vi "数字麦克风信号解析.vi"() -> ()   [LabVIEW 2024]
panel:
  in  "数值 2":i32=1
  out "长度":i32
  in  "数值":i32=400000
  out "文本":string
  out "波形图":i32[](graph)
  in  "路径":path=path "D:/Labviewworks/数字麦克风信号解析/采集数据文件/6060.log"
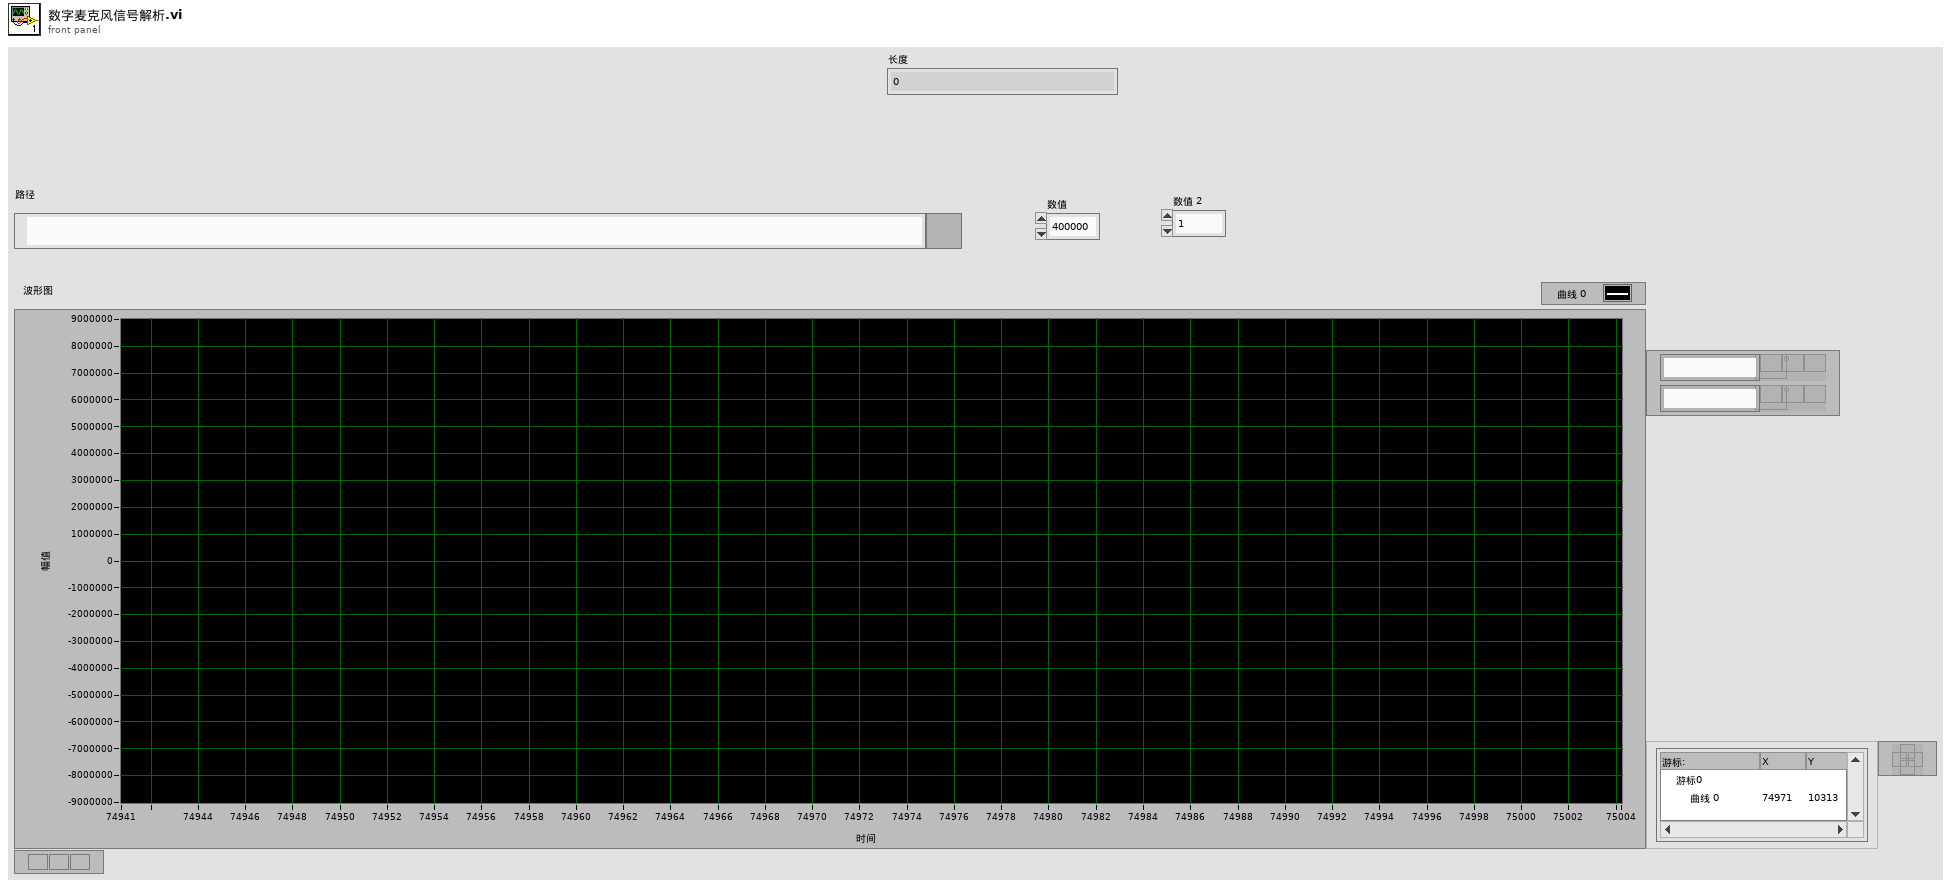
[diagram p1: front panel]
types:
  T1 = enum16{"open", "replace", "create", "open or create", "replace or create", "replace or create with confirmation"}
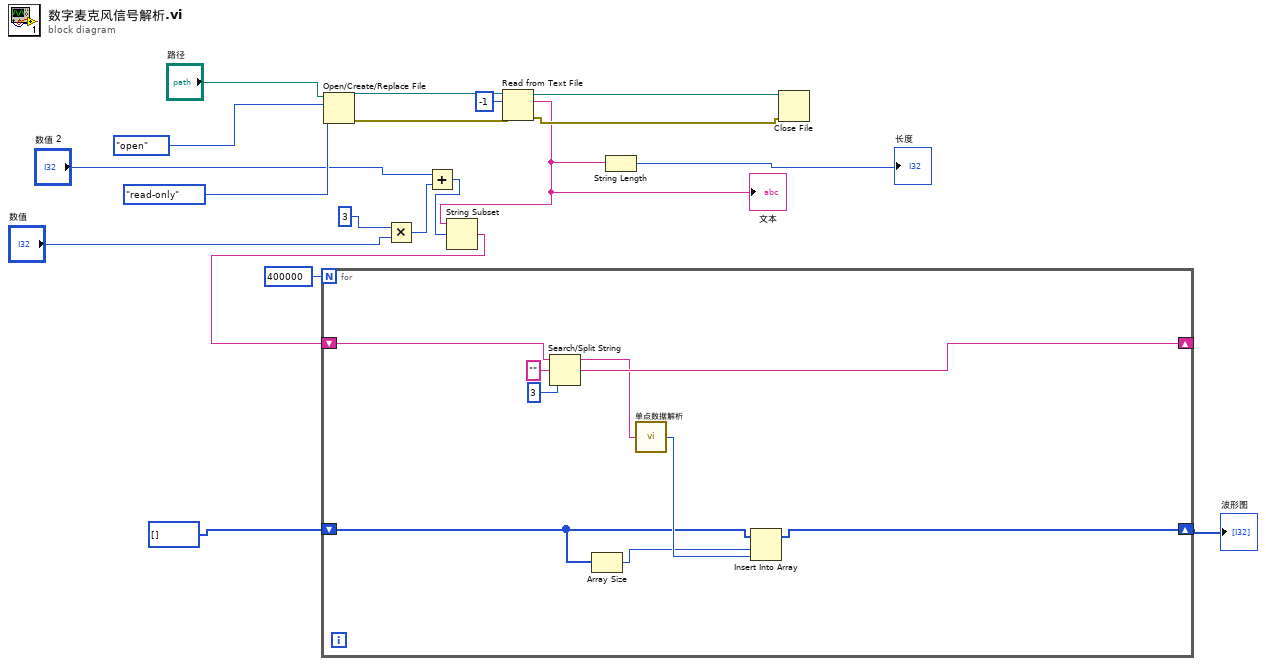
[diagram p0: block diagram]
diagram:
  n1 = Open/Create/Replace File(file path (use dialog)="路径", operation (0:open)=T1."open" ("操作(0:open)"), access (0:read/write)=enum16{"read/write", "read-only", "write-only"}."read-only" ("权限(0:read/write)")) -> (refnum out=w16:refnum<file>, error out=w15:errorcluster)  [unwired: 3 in, 1 out]
  n2 = Multiply(x=3, y="数值") -> (x*y=w5:i32)
  n3 = Add(x="数值 2", y=w5) -> (x+y=w3:i32)
  n4 = Read from Text File(file (use dialog)=w16, count=-1 ("计数"), error in=w15) -> (refnum out=w14:refnum<file>, text=w2:string, error out=w13:errorcluster)  [unwired: 1 in, 1 out]
  "文本" <- w2
  n5 = String Subset(string=w2, offset (0)=w3) -> (substring=w8:string)  [unwired: 1 in]
  n6 = for {
    N: 400000 -> [_]
    shift-right: [w25] -> _
    shift-left: w8 -> [w28]
    shift-right: [w20] -> w9
    shift-left: i32[] [] -> [w22]
    n7 = Search/Split String(string=w28, search string/char (-)="" ("搜索字符串/字符(-)"), offset (0)=3 ("偏移量(0)")) -> (substring before match=w24:string, match + rest of string=w25:string)  [unwired: 1 out]
    n8 = Array Size(array=w22) -> (size(s)=w21:i32)
    n9 = call "单点数据解析.vi"("字符串"=w24) -> ("*(类型 *) &x"=w23:i32)  [unwired: 4 in]
    n10 = Insert Into Array(array=w22, index=w21, new element=w23) -> (w20:i32[])
  }
  "波形图" <- w9
  n11 = String Length(string=w2) -> (length=→"长度":i32)
  n12 = Close File(refnum=w14, error in=w13) -> ()  [unwired: 2 out]
